vi "PCO_ImageDim.vi"(8 "error in":errorcluster caption="entrée d'erreur", 11 "configuration":T2={"exposure_time_s"=nan, "delay_time_s"=nan, "roi"={"x0"=18446744073709551615, "y0"=18446744073709551615, "x1"=18446744073709551615, "y1"=18446744073709551615}, "timestamp_mode"=65535, "pixelrate"=4294967295, "trigger_mode"=65535, "acquire_mode"=65535, "metadata_mode"=65535, "noisefilter_mode"=65535, "pixel_format"=4294967295, "binning"={"vert"=65535, "horz"=65535, "mode"=0}, "auto_exposure"={"region"=0, "min_exposure_s"=0.001, "max_exposure_s"=0.1}} {"auto_exposure"."region" items=["balanced", "center_based", "corner_based", "full", "custom"]; "binning"."mode" items=["sum", "average"]; "noisefilter_mode" items=["Undefined"=65535, "OFF"=0, "ON"=1]; "exposure_time_s" format="%#_6f"; "timestamp_mode" items=["Undefined"=65535, "OFF"=0, "Binary"=1, "Binary+ASCII"=2, "ASCII"=3]; "acquire_mode" items=["Undefined"=65535, "auto"=0, "external"=1, "external modulate"=2]; "trigger_mode" items=["Undefined"=65535, "auto sequence"=0, "software trigger"=1, "external exposure start & software trigger"=2, "external exposure control"=3, "external synchronized"=4, "fast external exposure control"=5, "external CDS control"=6, "slow external exposure control"=7, "external synchronized HDSDI"=258]; "metadata_mode" items=["Undefined"=65535, "OFF"=0, "ON"=1]}) -> (0 "error out":errorcluster caption="sortie d'erreur", 3 "Dimensions":dbl[](array[numeric]))   [LabVIEW 2026]
uses:
  pco.labview/camera/Controls/binning.ctl
  Controls/TypeDef_FGV.ctl
  pco.labview/camera/Camera.lvclass
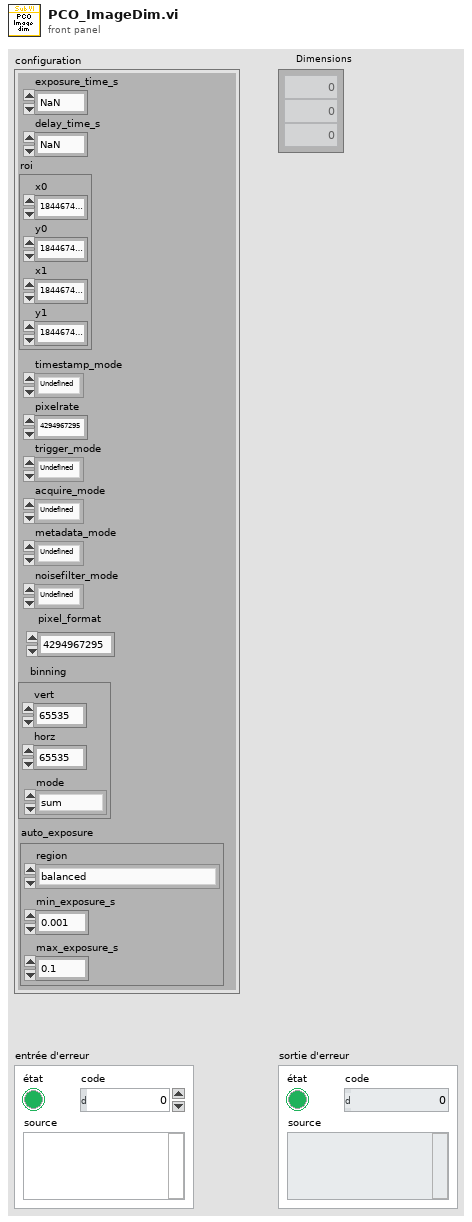
[diagram p1: front panel]
types:
  T1 = typedef "Camera.lvclass/binning.ctl" = cluster{"vert":u16, "horz":u16, "mode":u16}
  T2 = cluster{"exposure_time_s":dbl, "delay_time_s":dbl, "roi":cluster{"x0":u64, "y0":u64, "x1":u64, "y1":u64}, "timestamp_mode":u16, "pixelrate":u32, "trigger_mode":u16, "acquire_mode":u16, "metadata_mode":u16, "noisefilter_mode":u16, "pixel_format":u32, "binning":T1, "auto_exposure":cluster{"region":u16, "min_exposure_s":dbl, "max_exposure_s":dbl}}
  T3 = typedef "TypeDef_FGV.ctl" = enum16{"Initialize", "Write", "Read"}
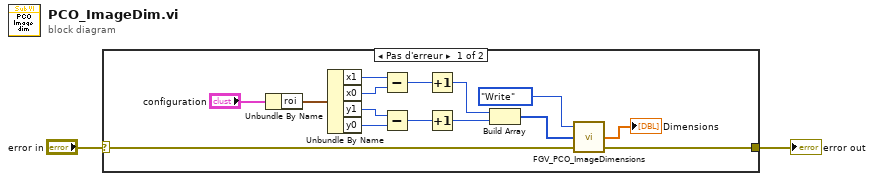
[diagram p0: block diagram]
diagram:
  n1 = case shown="Pas d'erreur" "error in" {
    selector: "error in" -> [w6 w18]
    tunnel: [w5 w18] -> w1
    frame No Error {
      n2 = Unbundle By Name("configuration") -> ("roi"=w11:cluster{"x0":u64, "y0":u64, "x1":u64, "y1":u64})
      n3 = Unbundle By Name(w11) -> ("x1"=w13:u64, "x0"=w12:u64, "y1"=w15:u64, "y0"=w14:u64)
      n4 = Subtract(x=w13, y=w12) -> (x-y=w16:u64)
      n5 = Subtract(x=w15, y=w14) -> (x-y=w17:u64)
      n6 = Increment(x=w16) -> (x+1=w9:u64)
      n7 = Increment(x=w17) -> (x+1=w8:u64)
      n8 = Build Array(w9, w8) -> (w7:u64[])
      n9 = call "FGV_PCO_ImageDimensions.vi"("error in"=w6, "Dimensions"=w7, "Action"=TypeDef_FGV."Write") -> ("error out"=w5:errorcluster, "Dimensions"=→"Dimensions":dbl[])  [unwired: 1 in]
    }
    frame Error {
    }
  }
  "error out" <- w1
